vi "pigeon_ver4_1.vi"() -> ()   [LabVIEW 2017]
uses:
  <vilib>/eio/EIONode/EIONode.xnode
  <vilib>/Platform/TimedLoop/XDataNode/XDataNode.xnode
  <vilib>/Platform/TimedLoop/XDataNode/nitl_modes.ctl
  <vilib>/Platform/TimedLoop/XDataNode/XDNodeRunTimeDep.lvlib
  <vilib>/Platform/TimedLoop/XDataNode/wakeup.ctl
  <vilib>/Platform/TimedLoop/XDataNode/timing_clust.ctl
  <vilib>/rvi/DataTransferAndStorage/Container/XNode/niFpgaContainer.xnode
  <vilib>/rvi/eio/common/nirviEmuTemplateMethod_errors.vi
  <vilib>/rvi/Memory/Memory_Emulation/nirvimemoryFastEmulation.vi
  <vilib>/rvi/Memory/Memory_Emulation/nirvimemoryEmulation.vi
  <vilib>/rvi/interface/RandomDataEmulation/nirviRandomDataFpgaReadWriteTemplate.vi
  <vilib>/rvi/Analysis/common/FxpNativeNode/niFpgaFxpNative.xnode
panel:
  out "ramp loop end?":bool=TRUE
  out "ctr":i16
  out "ramp start val":fxp<+,15,15>
  out "Numeric":i16
  in  "analog ramp on":bool
  out "AI2":i16
  in  "Tab Control":enum32{"pigeon"}(tab)
  in  "Emergency Stop":bool
  in  "AO7_pigeon":i16
  in  "AO7":i16
  in  "AO6":i16
  out "trigger AI1":bool
  in  "Tab Control 2":T1(tab)
  in  "square wave  on?":bool
  in  "square wave period":i32
  in  "IGBTswitch":bool caption="IGBT Switch circular"
  in  "Manual Override":bool
  in  "circular coil current":i16(slide) scale=0.0..32768.0
  in  "analog ramp period":i16
  in  "AO4":bool
  in  "analog wave shape":i16(ring) items=["Triangle", "Sawtooth", "Sin", ""]
  in  "analog ramp on  2":bool
  in  "End Current":fxp<+,16,16>
  out "approx rise time [uSec]":u32
  in  "Update Period (uSec)":u32=500
  in  "Points to Add (2^n - 1)":i16=3
  out "FIFO size":i16
  in  "AO0":i16
  in  "AO1":i16
  in  "AO2":i16
  in  "Run program":bool
  in  "halt processor":bool
  out "control flags":i8 format="%b"
  in  "host operation":i16
  in  "address":u16
  in  "data1":u16
  in  "data2":i32
  in  "repeat program":i32
  out "IP address":i16
  out "PMT1":i16=-4740
  out "ReA":i32
  out "RegB":i16
  out "RegC":i16
  out "exttrigger":bool=TRUE
  out "AI1":i16=161
  out "RegD":i16
  in  "AO4":i16
  in  "AO3":i16
  out "Connector0/AI0":i16
  in  "AO5":i16
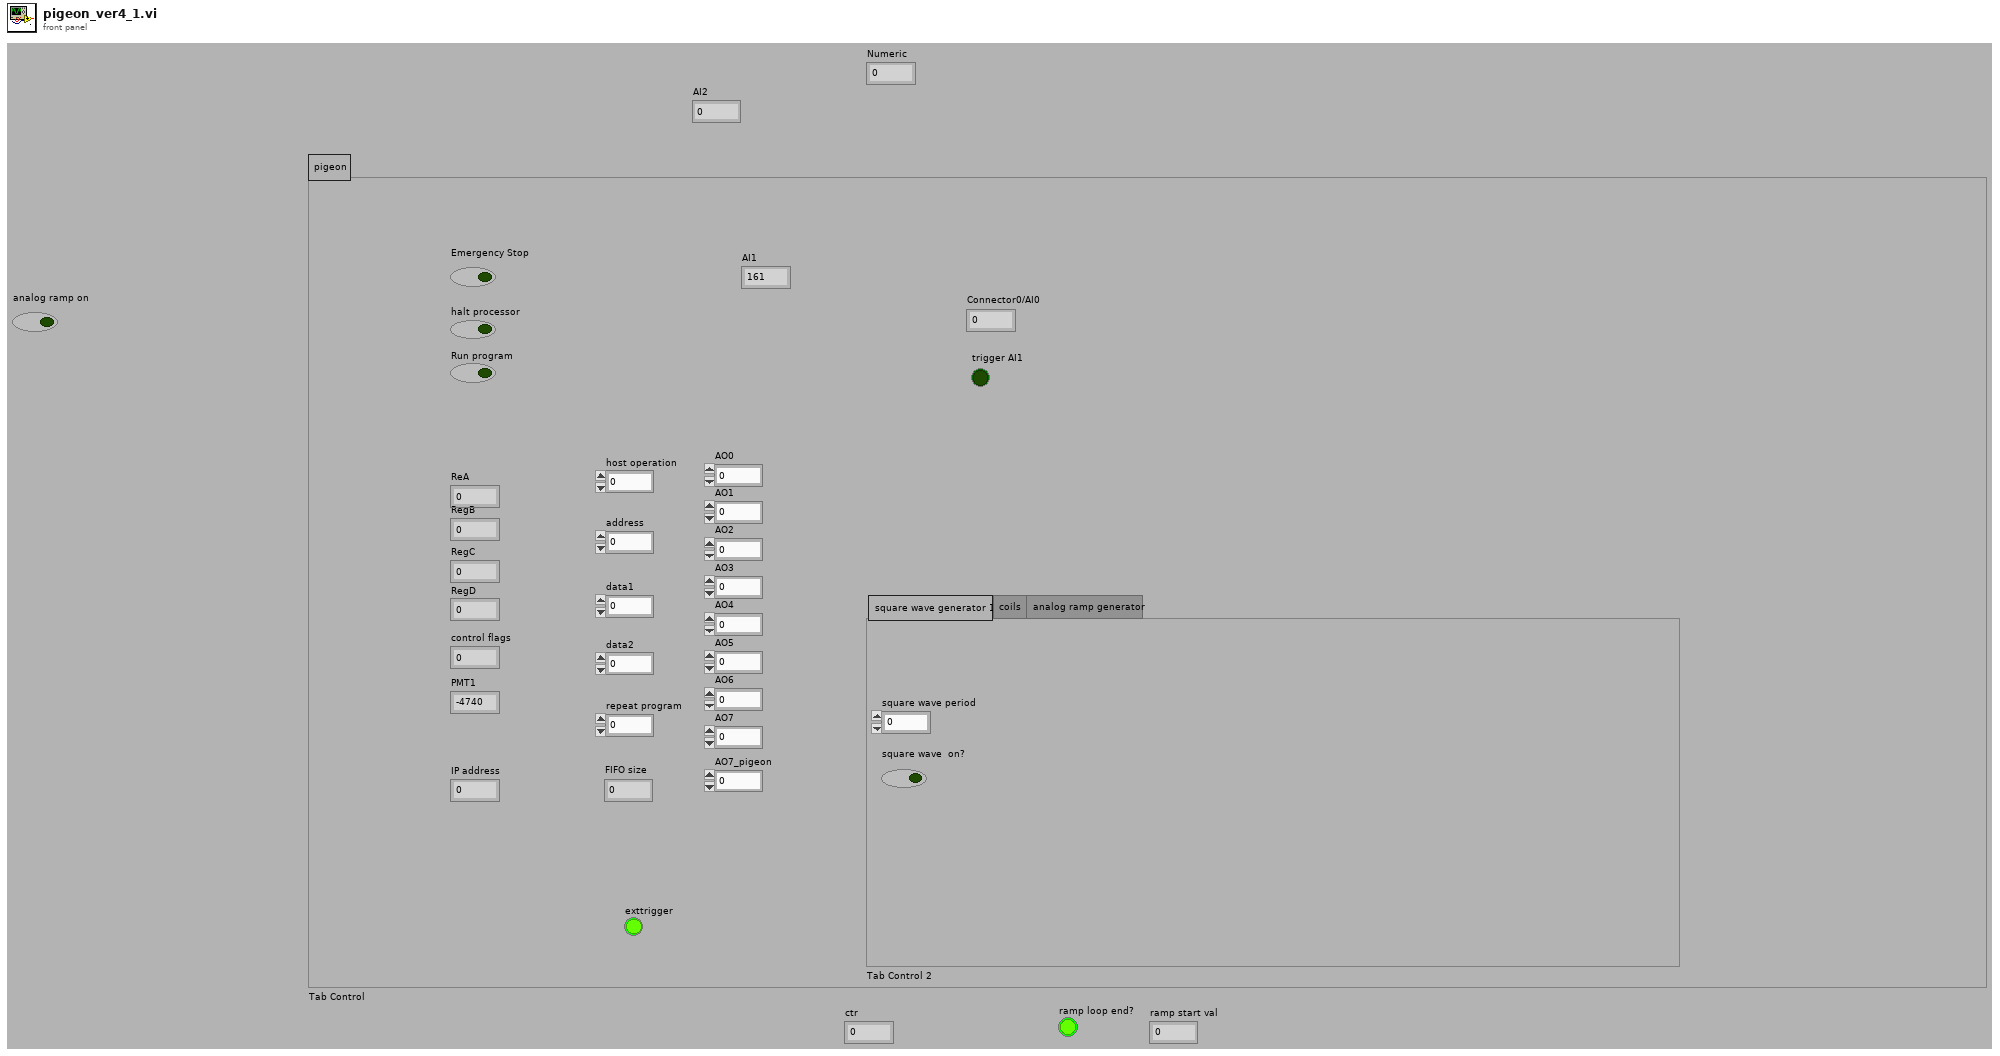
[diagram p1: front panel]
types:
  T1 = enum32{"square wave generator 1", "coils", "analog ramp generator"}
  T2 = typedef "XDNodeRunTimeDep.lvlib/timing_clust.ctl" = cluster{"Expected End [f-1]":u64, "Actual End [f-1]":u64, "Finished Late? [f-1]":bool, "Expected End [i-1]":u64, "Actual End [i-1]":u64, "Finished Late? [i-1]":bool, "Expected Start [i]":u64, "Actual Start [i]":u64, "Expected Start [f]":u64, "Actual Start [f]":u64, "Source Name":string, "Structure Name":string, "Period":i64, "Deadline":i64, "Offset":i64, "Start":i64, "Priority":i32, "Timeout":i32, "Mode":T3, "Wakeup Reason":T4, "Error":errorcluster, "Source Type":string, "Secondary Source Type":string, "Global End Time":u64, "Global Start Time":u64, "Frame Duration":u64, "Iteration Duration":u64, "Assigned CPU":i32, "I/O Scan Engine Mode":u32}
  T3 = typedef "XDNodeRunTimeDep.lvlib/nitl_modes.ctl" = enum32{"No Change", "Process missed periods, maintain original phase", "Discard missed periods, maintain original phase", "Process missed periods, ignore original phase", "Discard missed periods, ignore original phase"}
  T4 = typedef "XDNodeRunTimeDep.lvlib/wakeup.ctl" = enum32{"Normal", "Aborted", "Asynchronous wakeup", "Timing source error", "Timed loop error", "Timeout"}
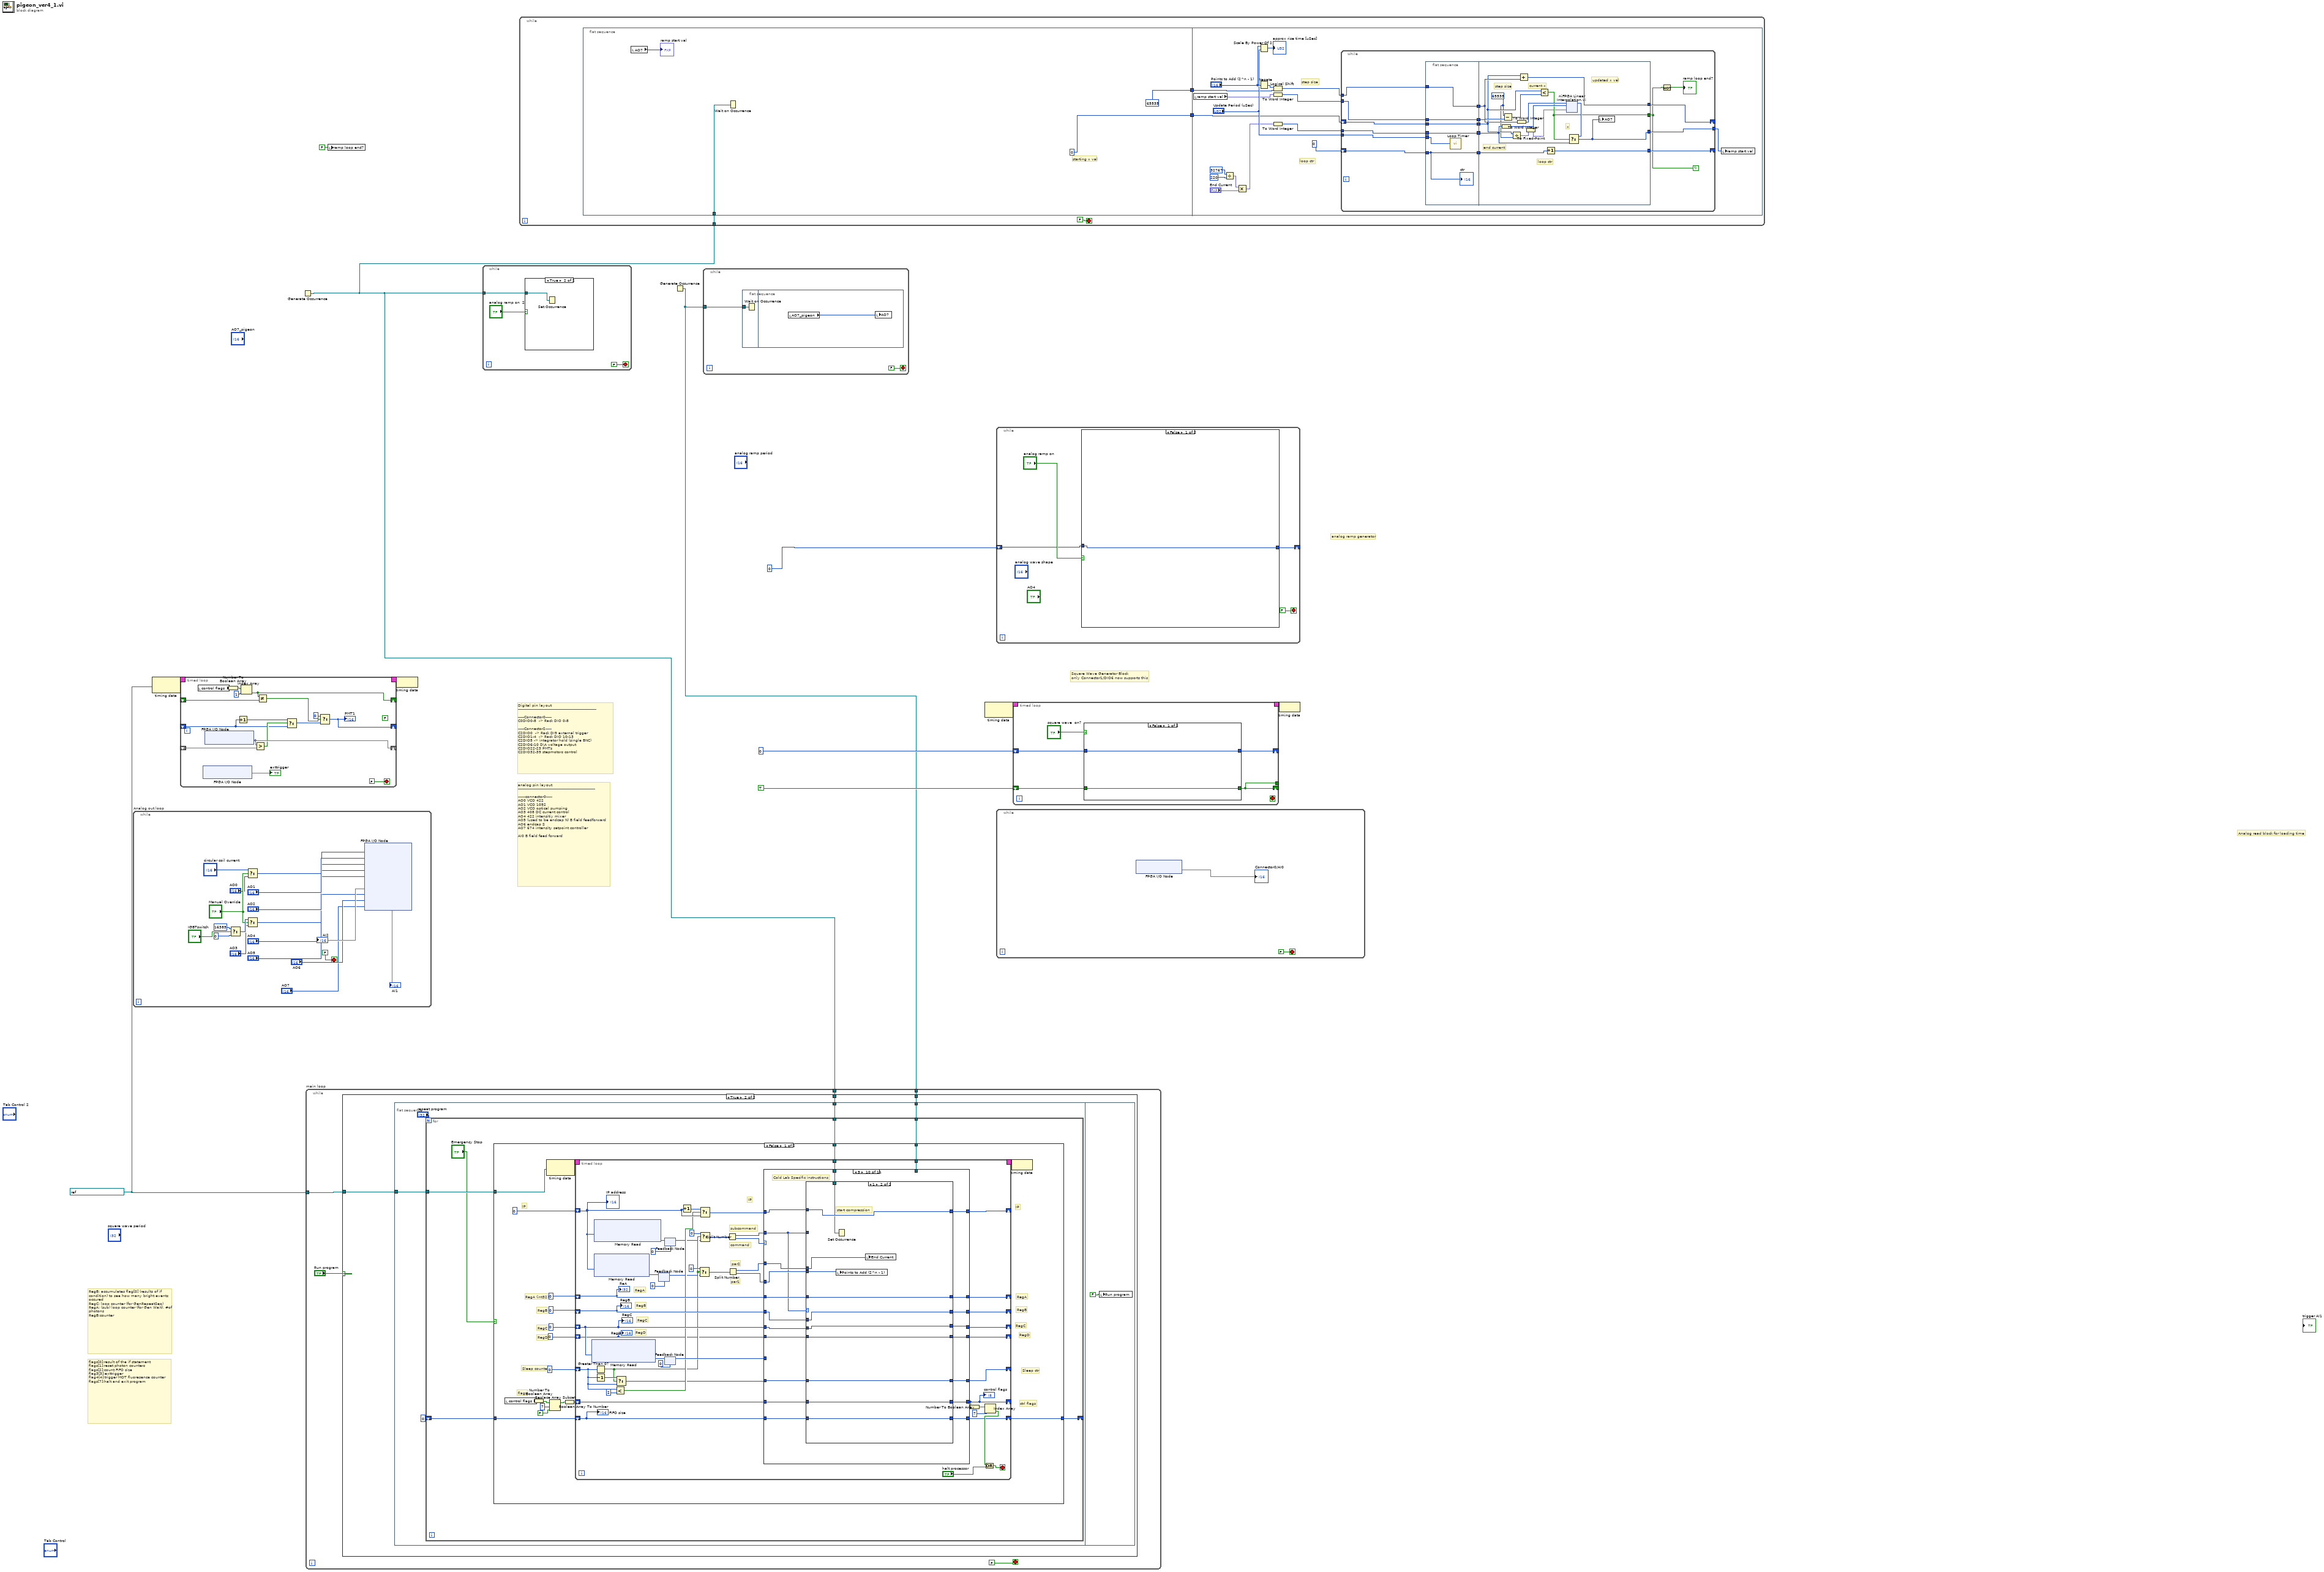
[diagram p0: block diagram]
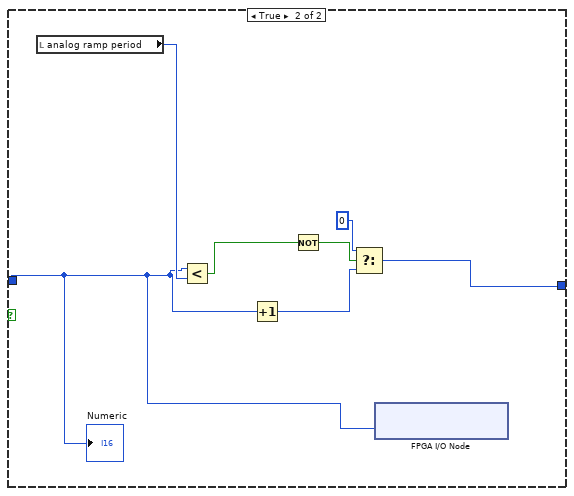
[diagram p3: hidden frame]
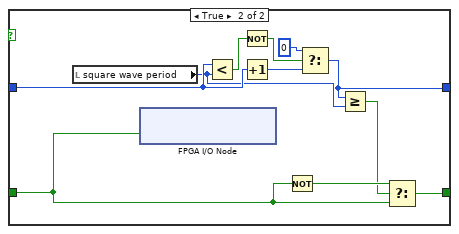
[diagram p4: hidden frame]
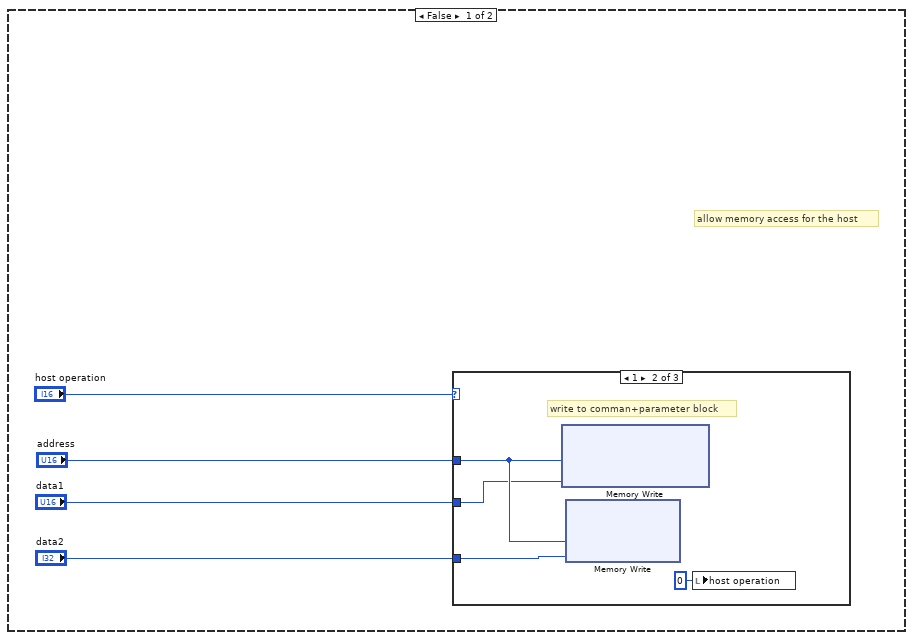
[diagram p5: hidden frame]
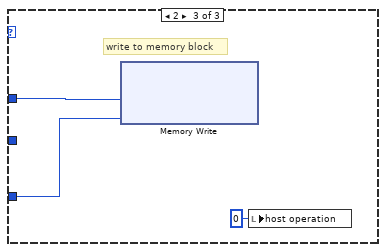
[diagram p7: hidden frame]
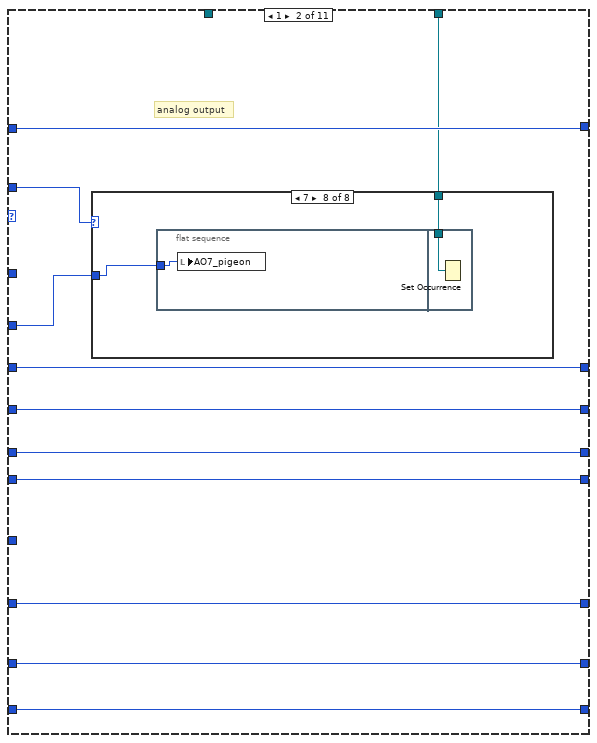
[diagram p9: hidden frame]
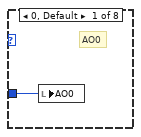
[diagram p10: hidden frame]
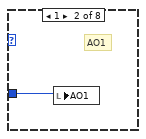
[diagram p11: hidden frame]
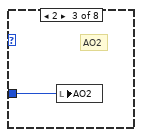
[diagram p12: hidden frame]
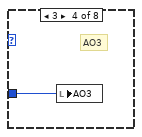
[diagram p13: hidden frame]
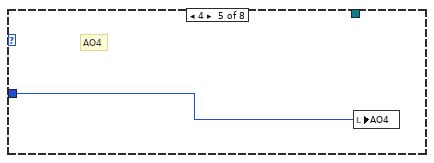
[diagram p14: hidden frame]
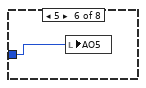
[diagram p15: hidden frame]
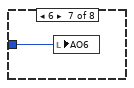
[diagram p16: hidden frame]
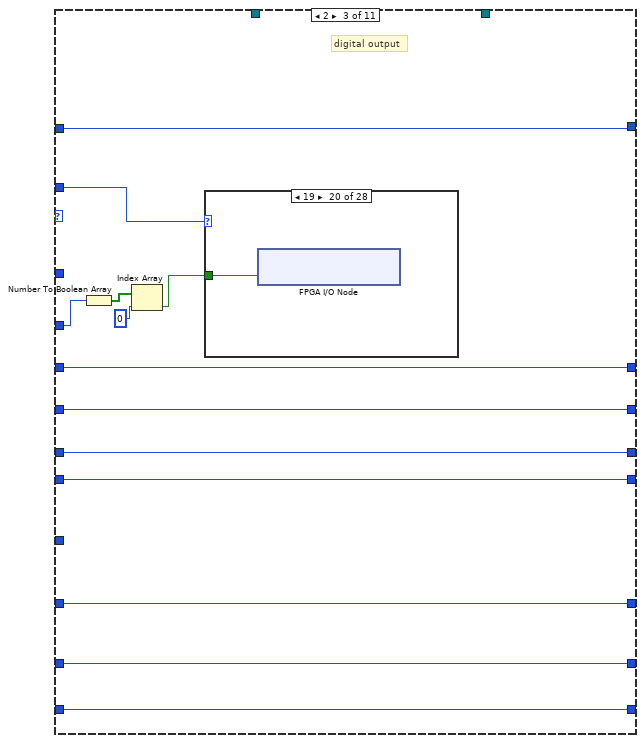
[diagram p17: hidden frame]
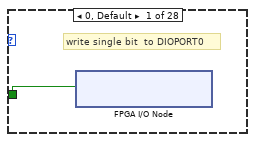
[diagram p18: hidden frame]
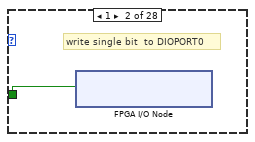
[diagram p19: hidden frame]
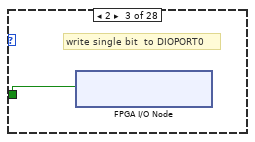
[diagram p20: hidden frame]
diagram:
  w9 = refnum<k21> "40 MHz Onboard Clock" ("FPGA Clock")
  # "analog ramp generator"
  # "Analog read block for loading time"
  # "Square Wave Generator Block\nonly Connector1/DIO6 now supports this"
  # "RegB: accumulates flag[0] (results of if condition) to see how many bright events occured\nRegC: loop counter (for GenRepeatSeq)\nRegA: (sub) loop counter (for Gen Wait), #of     photons \nRegB:counter"
  # "flags[0]:result of the if statement\nflags[1]:reset photon counters\nflags[2]:count FIFO size\nflag3[3]:exttrigger\nflag4[4]:trigger MOT fluoresence counter\nflags[7]:halt and exit program"
  # "Digital pin layout\n----------------------------------------------------------------\n\n-----Connector0-----\nC0DIO0-8  -> Rack DIO 0-8\n\n-----Connector2-----\nC2DIO0  -> Rack DI9 external trigger \nC2DIO1-4  -> Rack DIO 10-13\nC2DIO5 -> integrator hold (single BNC)\nC2DIO6-10 D\\A voltage output\nC2DIO22-23 PMTs\nC2DIO32-39 stepmotors control"
  # "analog pin layout\n---------------------------------------------------------------\n\n------connector0-----\nAO0 VCO 422\nAO1 VCO 1092\nAO2 VCO optical pumping\nAO3 408 DC current control\nAO4 422 intensitiy mixer\nAO5 (used to be endcap N) B field feedforward\nAO6 endcap S\nAO7 674 intensity setpoint controller\n\nAI0 B field feed forward"
  n1 = while "Analog out loop" {
    stop <- FALSE stop-if-true
    n2 = Select(t=i16 16385, s="IGBTswitch", f=i16 0) -> (s? t:f=w20:i16)
    n3 = Select(t="circular coil current", s="Manual Override", f="AO0") -> (s? t:f=w14:i16)
    n4 = Select(t=w20, s="Manual Override", f="AO3") -> (s? t:f=w19:i16)
    n5 = xnode "FPGA I/O Node"("Connector0/AO0"=w14, "Connector0/AO1"="AO1", "Connector0/AO2"="AO2", "Connector0/AO3"=w19, "Connector0/AO4"="AO4", "Connector0/AO5"="AO5", "Connector0/AO6"="AO6", "Connector0/AO7"="AO7") -> ("Connector0/AI1"=→"AI1", "Connector0/AI2"=→"AI2")  [unwired: 10 in, 10 out]
  }
  n6 = node-c288(w9) -> (w11:T2)
  n7 = timed-loop {
    timing: w11 -> [_]
    timing-out: [_] -> w10
    shift-right: [w44] -> _
    shift-left: _ -> [w33]
    shift-right: [w37] -> _
    shift-left: _ -> [w46]
    shift-right: [w39] -> _
    shift-left: _ -> [w40]
    stop <- FALSE stop-if-true
    (unwired) FALSE
    n8 = local read "control flags"() -> (w41:i8)
    n9 = xnode "FPGA I/O Node"() -> ("Connector2/DIO0"=→"exttrigger")  [unwired: 1 in, 1 out]
    n10 = xnode "FPGA I/O Node"() -> ("Connector0/DIO0"=w37)  [unwired: 1 in, 1 out]
    n11 = Number To Boolean Array(number=w41) -> (Boolean array=w42:bool[])
    n12 = Increment(x=w33) -> (x+1=w34:u16)
    n13 = Index Array(array=w42, index=1) -> (element=w39:bool)
    n14 = Greater?(x=w37, y=w46) -> (0:w36:bool)
    n15 = Not Equal?(x=w39, y=w40) -> (x != y?=w31:bool)
    n16 = Select(t=w34, s=w36, f=w33) -> (s? t:f=w45:u16)
    n17 = Select(t=u16 0, s=w31, f=w45) -> (s? t:f=w44:u16)
    "PMT1" <- w44
  }
  n18 = Generate Occurrence() -> (w2:refnum<k4>)
  n19 = local write "ramp loop end?"(FALSE ("ramp loop end?")) -> ()
  n20 = node-c288(w10) -> ()
  n21 = while {
    tunnel: w2 -> [w50]
    stop <- FALSE stop-if-true
    n22 = case shown="True" "analog ramp on  2" {
      tunnel: w50 -> [_ w52]
      frame False {
      }
      frame True {
        n23 = Set Occurrence(w52) -> ()
      }
    }
  }
  n24 = while {
    tunnel: w2 -> [w53]
    stop <- FALSE stop-if-true
    n25 = flat-sequence {
      tunnel: [u16 0] -> w55
      tunnel: [u16 65535 ("x")] -> w54
      tunnel: w53 -> [w57]
      tunnel: w55 -> [w65]
      tunnel: w54 -> [w66]
      frame #0 {
        # "starting x val"
        n26 = local read "AO7"() -> (→"ramp start val":i16)
        n27 = Wait on Occurrence(2:w57) -> ()  [unwired: 2 in, 1 out]
      }
      frame #1 {
        # "loop ctr"
        # "step size"
        n28 = local read "ramp start val"() -> (w62:fxp<+,15,15>)
        n29 = Divide(x=i16 32767, y=i16 220) -> (x/y=w75:fxp<+,16,16>)
        n30 = Multiply(x=w75, y="End Current") -> (x*y=w63:fxp<+,32,32>)
        n31 = Scale By Power Of 2(n="Points to Add (2^n - 1)", x="Update Period (uSec)") -> (x*2^n=→"approx rise time [uSec]":u32)
        n32 = Negate(x="Points to Add (2^n - 1)") -> (-x=w70:i16)
        n33 = Logical Shift(y=w70, x=w66) -> (x << y=w71:u16)
        n34 = To Word Integer(number=w62) -> (16bit integer=w73:i16)
        n35 = To Word Integer(number=w63) -> (16bit integer=w72:i16)
        n36 = while {
          tunnel: w71 -> [w81]
          tunnel: w73 -> [w93]
          tunnel: w72 -> [w92]
          shift-right: [w91] -> _
          shift-left: w65 -> [w80]
          tunnel: "Update Period (uSec)" -> [w90]
          shift-right: [w84] -> _
          shift-left: i16 0 -> [w82]
          tunnel: [w83] -> w64
          stop <- w79 continue-if-true
          n37 = flat-sequence {
            tunnel: w81 -> [w98]
            tunnel: [w98] -> w89
            tunnel: w93 -> [w97]
            tunnel: [w97] -> w88
            tunnel: w92 -> [w96]
            tunnel: [w96] -> w87
            tunnel: w80 -> [w95]
            tunnel: [w95] -> w86
            tunnel: w90 -> [w99]
            tunnel: w82 -> [w94]
            tunnel: [w94] -> w85
            tunnel: w89 -> [w107]
            tunnel: w88 -> [w115]
            tunnel: w87 -> [w105]
            tunnel: w86 -> [w103]
            tunnel: [w108] -> w79
            tunnel: [w109] -> w91
            tunnel: [w111] -> w84
            tunnel: w85 -> [w110]
            tunnel: [w100] -> w83
            frame #0 {
              n38 = call "Loop Timer"("Count(uSec)"=w99) -> ()  [unwired: 1 out]
              "ctr" <- w94
            }
            frame #1 {
              w101 = u16 65535 ("x")
              # "current x"
              # "end current"
              # "x"
              # "loop ctr"
              # "updated x val"
              # "step size"
              n39 = To Word Integer(number=w105) -> (16bit integer=w112:i16)
              n40 = Subtract(x=w101, y=w107) -> (x-y=w106:u16)
              n41 = Divide(x=w103, y=w101) -> (x/y=w102:fxp<+,16,0>)
              n42 = To Word Integer(number=w115) -> (16bit integer=w113:i16)
              n43 = Add(x=w103, y=w107) -> (x+y=w109:u16)
              n44 = To Fixed-Point(number=w102) -> (fixed-point=w104:fxp<+,16,0>)  [unwired: 1 in]
              n45 = Less?(x=w103, y=w106) -> (x < y?=w108:bool)
              n46 = Increment(x=w110) -> (x+1=w111:i16)
              n47 = xnode ("niFPGA Linear Interpolation.vi")("y0"=w113, "y1"=w112, "x"=w104) -> ("y"=w114:i16)
              n48 = Select(t=w114, s=w108, f=w105) -> (s? t:f=w100:i16)
              n49 = local write "AO7"(w100) -> ()
            }
          }
          n50 = Not(x=w79) -> (.not. x?=→"ramp loop end?":bool)
        }
        n51 = local write "ramp start val"(w64) -> ()
      }
    }
  }
  n52 = Generate Occurrence() -> (w1:refnum<k4>)
  n53 = while "main loop" {
    tunnel: w9 -> [w129]
    tunnel: w2 -> [w128]
    tunnel: w1 -> [w127]
    stop <- FALSE ("stop") stop-if-true
    n54 = case shown="True" "Run program" {
      tunnel: w129 -> [_ w145]
      tunnel: w128 -> [_ w144]
      tunnel: w127 -> [_ w143]
      frame False {
        # "allow memory access for the host"
        n55 = case shown="1" "host operation" {
          tunnel: "address" -> [_ w137 w142]
          tunnel: "data1" -> [_ w136 _]
          tunnel: "data2" -> [_ w139 w140]
          frame 0, Default {
          }
          frame 1 {
            # "write to comman+parameter block"
            n56 = xnode ("Memory Write")("Address"=w137, "Data"=w136) -> ()  [unwired: 1 in, 1 out]
            n57 = xnode ("Memory Write")("Address"=w137, "Data"=w139) -> ()  [unwired: 1 in, 1 out]
            n58 = local write "host operation"(i16 0 ("host operation")) -> ()
          }
          frame 2 {
            # "write to memory block"
            n59 = xnode ("Memory Write")("Address"=w142, "Data"=w140) -> ()  [unwired: 1 in, 1 out]
            n60 = local write "host operation"(i16 0 ("host operation")) -> ()
          }
        }
      }
      frame True {
        n61 = flat-sequence {
          tunnel: w145 -> [w149]
          tunnel: w144 -> [w147]
          tunnel: w143 -> [w146]
          frame #0 {
            n62 = for {
              N: "repeat program" -> [_]
              tunnel: w149 -> [w156]
              shift-right: [w154] -> _
              shift-left: i16 0 -> [w155]
              tunnel: w147 -> [w153]
              tunnel: w146 -> [w152]
              n63 = case shown="False" "Emergency Stop" {
                tunnel: w156 -> [w169 _]
                tunnel: w155 -> [w161 w633]
                tunnel: [w160 w633] -> w154
                tunnel: w153 -> [w158 _]
                tunnel: w152 -> [w157 _]
                frame False {
                  # "ctrl flags"
                  # "Sleep ctr"
                  # "RegD"
                  # "RegD"
                  # "Sleep counter"
                  # "flags"
                  # "RegC"
                  # "RegB"
                  # "RegA"
                  # "RegC"
                  # "RegB"
                  # "RegA (int32)"
                  # "IP"
                  # "IP"
                  n64 = local read "control flags"() -> (w164:i8)
                  n65 = Number To Boolean Array(number=w164) -> (Boolean array=w168:bool[])
                  n66 = node-c288(w169) -> (w175:T2)
                  n67 = Replace Array Subset(array=w168, new element=FALSE ("new element/subarray"), index=7) -> (w166:bool[])
                  n68 = Boolean Array To Number(Boolean array=w166) -> (number=w167:u8)
                  n69 = timed-loop {
                    timing: w175 -> [_]
                    timing-out: [_] -> w174
                    shift-right: [w212] -> _
                    shift-left: i16 0 -> [w195]
                    shift-right: [w208] -> _
                    shift-left: 0 -> [w204]
                    shift-right: [w220] -> _
                    shift-left: i16 0 -> [w211]
                    shift-right: [w219] -> _
                    shift-left: i16 0 -> [w203]
                    shift-right: [w209] -> _
                    shift-left: w167 -> [w210]
                    shift-right: [w202] -> _
                    shift-left: i16 0 -> [w193]
                    shift-right: [w184] -> w160
                    shift-left: w161 -> [w183]
                    shift-right: [w181] -> _
                    shift-left: i16 0 -> [w182]
                    tunnel: w158 -> [w177]
                    tunnel: w157 -> [w176]
                    stop <- w215 stop-if-true
                    # "RegD"
                    # "IP"
                    # "RegC"
                    # "RegB"
                    # "RegA"
                    # "par1"
                    # "par2"
                    # "subcommand"
                    # "command"
                    n70 = xnode ("Memory Read")("Address"=w203) -> ("Data"=w207:i16)  [unwired: 2 in, 2 out]
                    n71 = xnode ("Memory Read")("Address"=w195) -> ("Data"=w190:u16)  [unwired: 1 in, 1 out]
                    n72 = xnode ("Memory Read")("Address"=w195) -> ("Data"=w186:i32)  [unwired: 1 in, 1 out]
                    n73 = Greater Than 0?(x=w193) -> (x > 0?=w188:bool)
                    n74 = Decrement(x=w193) -> (x-1=w194:u32)
                    n75 = Less?(x=w193, y=u32 2) -> (x < y?=w192:bool)
                    n76 = Select(t=w194, s=w188, f=w193) -> (s? t:f=w191:u32)
                    n77 = feedback-in #1(w186) -> ()
                    n78 = feedback #1(u32 0 ("Data")) -> (w185:u32)
                    n79 = feedback-in #2(w207) -> ()
                    n80 = feedback #2(0) -> (w206:i32)
                    n81 = feedback-in #3(w190) -> ()
                    n82 = feedback #3(u16 0 ("Data")) -> (w187:u16)
                    n83 = Increment(x=w195) -> (x+1=w196:u16)
                    n84 = Select(t=0, s=w188, f=w185) -> (s? t:f=w199:u32)
                    n85 = Select(t=w196, s=w192, f=w195) -> (s? t:f=w201:u16)
                    n86 = Select(t=u16 0, s=w188, f=w187) -> (s? t:f=w200:u16)
                    n87 = Split Number(x=w200) -> (hi(x)=w221:u8, lo(x)=w222:u8)
                    n88 = Split Number(x=w199) -> (hi(x)=w213:u16, lo(x)=w214:u16)
                    n89 = case shown="9" w222 {
                      tunnel: w214 -> [_ w240 w257 _ w337 w457 w531 _ _ w591 _]
                      tunnel: w213 -> [_ _ _ _ w330 w456 w530 _ _ w592 _]
                      tunnel: w221 -> [_ w241 w265 w304 w338 w461 _ w549 _ w573 _]
                      tunnel: w204 -> [w230 w239 w264 w296 w336 w458 w535 w553 w569 w590 w620]
                      tunnel: [w230 w239 w264 w296 w333 w458 w535 w553 w569 w589 w620] -> w208
                      tunnel: w211 -> [w229 w238 w263 w295 w335 w459 w536 w552 w572 w588 w621]
                      tunnel: w203 -> [w228 w237 w262 w302 w334 w460 w537 w551 w571 w586 w622]
                      tunnel: [w229 w238 w263 w294 w332 w459 w536 w552 w572 w587 w621] -> w220
                      tunnel: [w228 w237 w262 w302 w331 w460 w537 w551 w571 w585 w622] -> w219
                      tunnel: [w226 w236 w261 w303 w326 w464 w529 w555 w570 w575 w619] -> w212
                      tunnel: w201 -> [w226 w236 w261 w303 w327 w464 _ w555 w570 w576 w619]
                      tunnel: [w227 w235 w260 w300 w328 w463 w528 w544 w566 w579 w625] -> w209
                      tunnel: w210 -> [w227 w235 w260 w301 w329 w462 w528 w543 w565 w580 w625]
                      tunnel: w206 -> [_ _ _ _ w320 w455 _ _ _ _ _]
                      tunnel: w191 -> [w225 w234 w255 w299 w325 w454 w527 w541 w562 w582 w626]
                      tunnel: [w225 w234 w255 w299 w324 w454 w527 w541 w562 w581 w626] -> w202
                      tunnel: w183 -> [w224 w233 w254 w298 w323 w453 w526 w540 w561 w577 w624]
                      tunnel: [w224 w233 w254 w298 w323 w453 w526 w539 w561 w578 w624] -> w184
                      tunnel: w182 -> [w223 w232 w253 w297 w322 w452 w525 w538 w560 w584 w623]
                      tunnel: [w223 w232 w253 w297 w321 w452 w525 w538 w560 w583 w623] -> w181
                      tunnel: w177 -> [_ _ _ _ _ _ _ _ _ w574 _]
                      tunnel: w176 -> [_ w231 _ _ _ _ _ _ _ _ _]
                      frame 0, Default {
                      }
                      frame 1 {
                        # "analog output"
                        n90 = case shown="7" w241 {
                          tunnel: w240 -> [w242 w243 w244 w245 w246 w247 w248 w250]
                          tunnel: w231 -> [_ _ _ _ _ _ _ w249]
                          frame 0, Default {
                            # "AO0"
                            n91 = local write "AO0"(w242) -> ()
                          }
                          frame 1 {
                            # "AO1"
                            n92 = local write "AO1"(w243) -> ()
                          }
                          frame 2 {
                            # "AO2"
                            n93 = local write "AO2"(w244) -> ()
                          }
                          frame 3 {
                            # "AO3"
                            n94 = local write "AO3"(w245) -> ()
                          }
                          frame 4 {
                            # "AO4"
                            n95 = local write "AO4"(w246) -> ()
                          }
                          frame 5 {
                            n96 = local write "AO5"(w247) -> ()
                          }
                          frame 6 {
                            n97 = local write "AO6"(w248) -> ()
                          }
                          frame 7 {
                            n98 = flat-sequence {
                              tunnel: w250 -> [w251]
                              tunnel: w249 -> [w252]
                              frame #0 {
                                n99 = local write "AO7_pigeon"(w251) -> ()
                              }
                              frame #1 {
                                n100 = Set Occurrence(w252) -> ()
                              }
                            }
                          }
                        }
                      }
                      frame 2 {
                        # "digital output"
                        n101 = Number To Boolean Array(number=w257) -> (Boolean array=w258:bool[])
                        n102 = Index Array(array=w258, index=0) -> (element=w256:bool)
                        n103 = case shown="19" w265 {
                          tunnel: w256 -> [w266 w267 w268 w269 w270 w271 w272 w273 w274 w275 w276 w277 w278 w279 w280 w281 w282 w283 w284 w285 w286 w287 w288 w289 w290 w291 w292 w293]
                          frame 0, Default {
                            # "write single bit  to DIOPORT0"
                            n104 = xnode "FPGA I/O Node"("Connector1/DIO0"=w266) -> ()  [unwired: 1 in, 1 out]
                          }
                          frame 1 {
                            # "write single bit  to DIOPORT0"
                            n105 = xnode "FPGA I/O Node"("Connector1/DIO1"=w267) -> ()  [unwired: 1 in, 1 out]
                          }
                          frame 2 {
                            # "write single bit  to DIOPORT0"
                            n106 = xnode "FPGA I/O Node"("Connector1/DIO2"=w268) -> ()  [unwired: 1 in, 1 out]
                          }
                          frame 3 {
                            # "write single bit  to DIOPORT0"
                            n107 = xnode "FPGA I/O Node"("Connector1/DIO3"=w269) -> ()  [unwired: 1 in, 1 out]
                          }
                          frame 4 {
                            # "write single bit  to DIOPORT0"
                            n108 = xnode "FPGA I/O Node"("Connector1/DIO4"=w270) -> ()  [unwired: 1 in, 1 out]
                          }
                          frame 5 {
                            # "write single bit  to DIOPORT0"
                            n109 = xnode "FPGA I/O Node"("Connector1/DIO5"=w271) -> ()  [unwired: 1 in, 1 out]
                          }
                          frame 6 {
                            # "write single bit  to DIOPORT0"
                            n110 = xnode "FPGA I/O Node"("Connector1/DIO6"=w272) -> ()  [unwired: 1 in, 1 out]
                          }
                          frame 7 {
                            # "write single bit  to DIOPORT0"
                            n111 = xnode "FPGA I/O Node"("Connector1/DIO7"=w273) -> ()  [unwired: 1 in, 1 out]
                          }
                          frame 8 {
                            # "write single bit  to DIOPORT0"
                            n112 = xnode "FPGA I/O Node"("Connector1/DIO8"=w274) -> ()  [unwired: 1 in, 1 out]
                          }
                          frame 9 {
                            n113 = xnode "FPGA I/O Node"("Connector1/DIO9"=w275) -> ()  [unwired: 1 in, 1 out]
                          }
                          frame 10 {
                            n114 = xnode "FPGA I/O Node"("Connector1/DIO10"=w276) -> ()  [unwired: 1 in, 1 out]
                          }
                          frame 11 {
                            n115 = xnode "FPGA I/O Node"("Connector1/DIO11"=w277) -> ()  [unwired: 1 in, 1 out]
                          }
                          frame 12 {
                            n116 = xnode "FPGA I/O Node"("Connector1/DIO12"=w278) -> ()  [unwired: 1 in, 1 out]
                          }
                          frame 13 {
                            n117 = xnode "FPGA I/O Node"("Connector1/DIO13"=w279) -> ()  [unwired: 1 in, 1 out]
                          }
                          frame 14 {
                            n118 = xnode "FPGA I/O Node"("Connector1/DIO14"=w280) -> ()  [unwired: 1 in, 1 out]
                          }
                          frame 15 {
                            n119 = xnode "FPGA I/O Node"("Connector1/DIO15"=w281) -> ()  [unwired: 1 in, 1 out]
                          }
                          frame 16 {
                            n120 = xnode "FPGA I/O Node"("Connector1/DIO16"=w282) -> ()  [unwired: 1 in, 1 out]
                          }
                          frame 17 {
                            n121 = xnode "FPGA I/O Node"("Connector1/DIO17"=w283) -> ()  [unwired: 1 in, 1 out]
                          }
                          frame 18 {
                            n122 = xnode "FPGA I/O Node"("Connector1/DIO18"=w284) -> ()  [unwired: 1 in, 1 out]
                          }
                          frame 19 {
                            n123 = xnode "FPGA I/O Node"("Connector1/DIO19"=w285) -> ()  [unwired: 1 in, 1 out]
                          }
                          frame 20 {
                            n124 = xnode "FPGA I/O Node"("Connector2/DIO12"=w286) -> ()  [unwired: 1 in, 1 out]
                          }
                          frame 21 {
                            n125 = xnode "FPGA I/O Node"("Connector2/DIO17"=w287) -> ()  [unwired: 1 in, 1 out]
                          }
                          frame 22 {
                            n126 = xnode "FPGA I/O Node"("Connector2/DIO19"=w288) -> ()  [unwired: 1 in, 1 out]
                          }
                          frame 23 {
                            n127 = xnode "FPGA I/O Node"("Connector2/DIO18"=w289) -> ()  [unwired: 1 in, 1 out]
                          }
                          frame 24 {
                            n128 = xnode "FPGA I/O Node"("Connector2/DIO21"=w290) -> ()  [unwired: 1 in, 1 out]
                          }
                          frame 25 {
                            n129 = xnode "FPGA I/O Node"("Connector2/DIO24"=w291) -> ()  [unwired: 1 in, 1 out]
                          }
                          frame 26 {
                            n130 = xnode "FPGA I/O Node"("Connector2/DIO25"=w292) -> ()  [unwired: 1 in, 1 out]
                          }
                          frame 27 {
                            n131 = xnode "FPGA I/O Node"("Connector2/DIO20"=w293) -> ()  [unwired: 1 in, 1 out]
                          }
                        }
                      }
                      frame 3 {
                        # "photon counting"
                        n132 = case shown="3" w304 {
                          tunnel: [w305 w307 w319] -> w294
                          tunnel: w295 -> [w305 w308 w319]
                          tunnel: w301 -> [w306 w310 w317]
                          tunnel: [w306 w310 w316] -> w300
                          frame 2, Default {
                          }
                          frame 1 {
                            # "PMT1"
                            n133 = local read "PMT1"() -> (w309:i16)
                            n134 = Add(x=w309, y=w308) -> (x+y=w307:u16)
                          }
                          frame 3 {
                            # "Reset  photon counter"
                            # "make a Not gate of flag(1)"
                            n135 = Number To Boolean Array(number=w317) -> (Boolean array=w314:bool[])
                            n136 = Index Array(array=w314, index=1) -> (element=w312:bool)
                            n137 = Not(x=w312) -> (.not. x?=w311:bool)
                            n138 = Replace Array Subset(array=w314, new element=w311, index=1) -> (w315:bool[])
                            n139 = Boolean Array To Number(Boolean array=w315) -> (number=w316:u8)
                          }
                        }
                      }
                      frame 4 {
                        # "registers operation"
                        n140 = case shown="7" w338 {
                          tunnel: w337 -> [w344 w354 w361 _ _ _ _ w403 _ _ w430 w443]
                          tunnel: w336 -> [_ w353 w360 w367 w375 w383 w387 w408 w419 w425 w435 w448]
                          tunnel: w335 -> [w347 _ w359 w366 w377 w382 w395 w407 w418 w421 w433 w446]
                          tunnel: w334 -> [w346 w352 _ w369 w376 _ w388 w406 w417 w424 w434 w447]
                          tunnel: [w343 w353 w360 w367 w374 w383 w387 w408 w419 w425 w435 w448] -> w333
                          tunnel: [w347 w354 w359 w366 w377 w382 w394 w407 w418 w423 w433 w446] -> w332
                          tunnel: [w346 w352 w361 w368 w376 w382 w388 w406 w417 w424 w434 w447] -> w331
                          tunnel: w330 -> [w345 _ _ _ _ _ _ w404 _ _ _ w442]
                          tunnel: w329 -> [w342 w351 w358 w365 w373 w381 w389 w405 w416 w428 w438 w451]
                          tunnel: [w342 w351 w358 w365 w373 w381 w389 w405 w416 w428 w438 w451] -> w328
                          tunnel: w327 -> [w341 w350 w357 w364 w372 w380 w386 w397 w411 w427 w437 w450]
                          tunnel: [w341 w350 w357 w364 w372 w380 w386 w400 w414 w427 w437 w450] -> w326
                          tunnel: w325 -> [w340 w349 w356 w363 w371 w379 w385 _ _ w426 w436 w449]
                          tunnel: [w340 w349 w356 w363 w371 w379 w385 w401 w409 w426 w436 w449] -> w324
                          tunnel: w322 -> [w339 w348 w355 w362 w370 w378 w384 w396 w410 w420 _ w441]
                          tunnel: [w339 w348 w355 w362 w370 w378 w384 w396 w410 w420 w431 w440] -> w321
                          tunnel: w320 -> [_ _ _ _ _ _ _ _ w409 _ _ _]
                          frame 0, Default {
                            # "Set par1,2 to RegA"
                            n141 = Join Numbers(hi=w345, lo=w344) -> ((hi.lo)=w343:u32)
                          }
                          frame 1 {
                            # "Set par1 to RegB"
                          }
                          frame 2 {
                            # "Set par1 to RegC"
                          }
                          frame 3 {
                            # "increase RegC by 1"
                            n142 = Increment(x=w369) -> (x+1=w368:u16)
                          }
                          frame 4 {
                            # "increase RegA by 1"
                            n143 = Increment(x=w375) -> (x+1=w374:u32)
                          }
                          frame 5 {
                            # "Set regC to regB"
                          }
                          frame 6 {
                            # "regB<-regB+flags[0]"
                            n144 = Number To Boolean Array(number=w389) -> (Boolean array=w393:bool[])
                            n145 = Index Array(array=w393, index=0) -> (element=w391:bool)
                            n146 = Boolean To (0,1)(Boolean=w391) -> (0, 1=w390:i16)
                            n147 = Add(x=w390, y=w395) -> (x+y=w394:u16)
                          }
                          frame 7 {
                            # "Sleep counter = [par1 par2]"
                            n148 = Join Numbers(hi=w404, lo=w403) -> ((hi.lo)=w401:u32)
                            n149 = Greater?(x=w401, y=u32 0) -> (0:w399:bool)
                            n150 = Decrement(x=w397) -> (x-1=w398:u16)
                            n151 = Select(t=w398, s=w399, f=w397) -> (s? t:f=w400:u16)
                          }
                          frame 11 {
                            # "Sleep counter =par1* memory Block[RegC]"
                            n152 = Greater?(x=w409, y=u32 0) -> (0:w413:bool)
                            n153 = Decrement(x=w411) -> (x-1=w412:u16)
                            n154 = Select(t=w412, s=w413, f=w411) -> (s? t:f=w414:u16)
                          }
                          frame 8 {
                            # "RegB=RegB+ RegA(lo)"
                            n155 = Split Number(x=w425) -> (lo(x)=w422:u16)  [unwired: 1 out]
                            n156 = Add(x=w422, y=w421) -> (x+y=w423:u16)
                          }
                          frame 9 {
                            # "RegD<-AI1+par1"
                            n157 = To Word Integer(number=w430) -> (16bit integer=w429:i16)
                            n158 = local read "AI1"() -> (w432:i16)
                            n159 = Add(x=w429, y=w432) -> (x+y=w431:i16)
                          }
                          frame 10 {
                            # "RegD<-RegD*2^par1*par2"
                            n160 = To Word Integer(number=w442) -> (16bit integer=w444:i16)
                            n161 = To Word Integer(number=w443) -> (16bit integer=w445:i16)
                            n162 = Multiply(x=w444, y=w441) -> (x*y=w439:i16)
                            n163 = Scale By Power Of 2(n=w445, x=w439) -> (x*2^n=w440:i16)
                          }
                        }
                      }
                      frame 5 {
                        # "If statement"
                        n164 = case shown="4" w461 {
                          tunnel: [w474 w482 w490 w498 w508 w511 w519] -> w463
                          tunnel: w462 -> [w473 w481 w489 w497 w507 w512 w520]
                          tunnel: w456 -> [w467 _ _ _ _ _ _]
                          tunnel: w460 -> [_ _ w485 w492 _ _ _]
                          tunnel: w459 -> [_ w476 _ w491 _ _ _]
                          tunnel: w458 -> [w468 _ _ _ _ w509 w517]
                          tunnel: w457 -> [w466 w475 w484 _ _ w510 _]
                          tunnel: w455 -> [_ _ _ _ _ _ w524]
                          frame 0, Default {
                            # "The if regA =  [par1,par2]"
                            n165 = Number To Boolean Array(number=w473) -> (Boolean array=w471:bool[])
                            n166 = Join Numbers(hi=w467, lo=w466) -> ((hi.lo)=w465:u32)
                            n167 = Equal?(x=w465, y=w468) -> (x = y?=w469:bool)
                            n168 = Replace Array Subset(array=w471, new element=w469, index=0) -> (w470:bool[])
                            n169 = Boolean Array To Number(Boolean array=w470) -> (number=w474:u8)
                          }
                          frame 1 {
                            # "The if  regB >  par1"
                            n170 = Number To Boolean Array(number=w481) -> (Boolean array=w479:bool[])
                            n171 = Greater?(x=w476, y=w475) -> (0:w477:bool)
                            n172 = Replace Array Subset(array=w479, new element=w477, index=0) -> (w478:bool[])
                            n173 = Boolean Array To Number(Boolean array=w478) -> (number=w482:u8)
                          }
                          frame 2 {
                            # "The if  regC=  par1"
                            n174 = Number To Boolean Array(number=w489) -> (Boolean array=w487:bool[])
                            n175 = Equal?(x=w484, y=w485) -> (x = y?=w483:bool)
                            n176 = Replace Array Subset(array=w487, new element=w483, index=0) -> (w486:bool[])
                            n177 = Boolean Array To Number(Boolean array=w486) -> (number=w490:u8)
                          }
                          frame 3 {
                            # "The if  regB> regC"
                            n178 = Number To Boolean Array(number=w497) -> (Boolean array=w495:bool[])
                            n179 = Greater?(x=w491, y=w492) -> (0:w493:bool)
                            n180 = Replace Array Subset(array=w495, new element=w493, index=0) -> (w494:bool[])
                            n181 = Boolean Array To Number(Boolean array=w494) -> (number=w498:u8)
                          }
                          frame 4 {
                            w503 = 3 ("index")
                            # "external trigger rising edge"
                            n182 = Number To Boolean Array(number=w507) -> (Boolean array=w504:bool[])
                            n183 = local read "exttrigger"() -> (w500:bool)
                            n184 = Index Array(array=w504, index=w503) -> (element=w502:bool)
                            n185 = Not(x=w502) -> (.not. x?=w501:bool)
                            n186 = And(x=w500, y=w501) -> (x .and. y?=w499:bool)
                            n187 = Replace Array Subset(array=w504, new element #1=w499, index #1=0 ("index"), new element #2=w500, index #2=w503) -> (w505:bool[])
                            n188 = Boolean Array To Number(Boolean array=w505) -> (number=w508:u8)
                          }
                          frame 5 {
                            # "The if  regA >  par1"
                            n189 = Number To Boolean Array(number=w512) -> (Boolean array=w515:bool[])
                            n190 = Greater?(x=w509, y=w510) -> (0:w513:bool)
                            n191 = Replace Array Subset(array=w515, new element=w513, index=0) -> (w514:bool[])
                            n192 = Boolean Array To Number(Boolean array=w514) -> (number=w511:u8)
                          }
                          frame 6 {
                            # "The if  regA == memoryBlock(regC)"
                            n193 = Number To Boolean Array(number=w520) -> (Boolean array=w522:bool[])
                            n194 = Equal?(x=w517, y=w524) -> (x = y?=w518:bool)
                            n195 = Replace Array Subset(array=w522, new element=w518, index=0) -> (w521:bool[])
                            n196 = Boolean Array To Number(Boolean array=w521) -> (number=w519:u8)
                          }
                        }
                      }
                      frame 6 {
                        # "condition (flags[0]) goto\nuse par1=par2 for normal goto"
                        n197 = Number To Boolean Array(number=w528) -> (Boolean array=w534:bool[])
                        n198 = Index Array(array=w534, index=0) -> (element=w532:bool)
                        n199 = Select(t=w531, s=w532, f=w530) -> (s? t:f=w529:u16)
                      }
                      frame 7 {
                        w542 = 2 ("index")
                        # "make a Not gate of flag(2)"
                        # "push  to FIFO"
                        n200 = case shown="4" w549 {
                          tunnel: w553 -> [w556 _ _ _]
                          tunnel: w552 -> [_ w557 _ _]
                          tunnel: w551 -> [_ _ w558 _]
                          tunnel: [w556 w557 w558 w559] -> w550
                          frame 0, Default {
                            # "push RegA"
                          }
                          frame 1 {
                            # "push RegB"
                          }
                          frame 2 {
                            # "push RegC"
                          }
                          frame 4 {
                            n201 = local read "AI1"() -> (w559:i16)
                          }
                        }
                        n202 = Number To Boolean Array(number=w543) -> (Boolean array=w547:bool[])
                        n203 = Index Array(array=w547, index=w542) -> (element=w546:bool)
                        n204 = Not(x=w546) -> (.not. x?=w545:bool)
                        n205 = Replace Array Subset(array=w547, new element=w545, index=w542) -> (w548:bool[])
                        n206 = Increment(x=w540) -> (x+1=w539:i16)
                        n207 = Boolean Array To Number(Boolean array=w548) -> (number=w544:u8)
                        n208 = xnode ("FIFO Write")("Element"=w550, "Timeout"=0) -> ()  [unwired: 1 in, 2 out]
                      }
                      frame 8 {
                        # "Stop and reset program"
                        n209 = Number To Boolean Array(number=w565) -> (Boolean array=w568:bool[])
                        n210 = Replace Array Subset(array=w568, new element=TRUE ("new element/subarray"), index=7) -> (w567:bool[])
                        n211 = Boolean Array To Number(Boolean array=w567) -> (number=w566:u8)
                      }
                      frame 9 {
                        # "Cold Lab Specific instructions"
                        n212 = case shown="1" w573 {
                          tunnel: w592 -> [w605 w610]
                          tunnel: w591 -> [w604 w609]
                          tunnel: w590 -> [w601 w611]
                          tunnel: [w601 w611] -> w589
                          tunnel: w588 -> [w600 w612]
                          tunnel: [w600 w612] -> w587
                          tunnel: w586 -> [w599 w613]
                          tunnel: [w599 w613] -> w585
                          tunnel: w584 -> [w598 w614]
                          tunnel: [w598 w614] -> w583
                          tunnel: w582 -> [w597 w615]
                          tunnel: [w597 w615] -> w581
                          tunnel: w580 -> [w596 w616]
                          tunnel: [w596 w616] -> w579
                          tunnel: [w595 w617] -> w578
                          tunnel: w577 -> [w595 w617]
                          tunnel: w576 -> [w594 w608]
                          tunnel: [w594 w608] -> w575
                          tunnel: w574 -> [_ w607]
                          tunnel: w573 -> [w593 _]
                          frame 0, Default {
                            # "Run Square wave generator"
                            n213 = Greater?(x=w593, y=u8 0) -> (0:w602:bool)
                            n214 = Join Numbers(hi=w605, lo=w604) -> ((hi.lo)=w606:u32)
                            n215 = local write "square wave  on?"(w602) -> ()
                            n216 = local write "square wave period"(w606) -> ()
                          }
                          frame 1 {
                            # "start compression"
                            n217 = Set Occurrence(w607) -> ()
                            n218 = local write "Points to Add (2^n - 1)"(w609) -> ()
                            n219 = local write "End Current"(w610) -> ()
                          }
                        }
                      }
                      frame 10 {
                        n220 = local write "trigger AI1"(TRUE) -> ()
                      }
                    }
                    "control flags" <- w209
                    n221 = Number To Boolean Array(number=w209) -> (Boolean array=w218:bool[])
                    n222 = Index Array(array=w218, index=7) -> (element=w216:bool)
                    n223 = Or(x=w216, y="halt processor") -> (x .or. y?=w215:bool)
                    "IP address" <- w195
                    "ReA" <- w204
                    "RegB" <- w211
                    "RegC" <- w203
                    "FIFO size" <- w183
                    "RegD" <- w182
                  }
                  n224 = node-c288(w174) -> ()
                }
                frame True {
                }
              }
            }
          }
          frame #1 {
            n225 = local write "Run program"(FALSE ("Run program")) -> ()
          }
        }
      }
    }
  }
  n226 = while {
    tunnel: w1 -> [w636]
    stop <- FALSE stop-if-true
    n227 = flat-sequence {
      tunnel: w636 -> [w637]
      frame #0 {
        n228 = Wait on Occurrence(2:w637) -> ()  [unwired: 2 in, 1 out]
      }
      frame #1 {
        n229 = local read "AO7_pigeon"() -> (w638:i16)
        n230 = local write "AO7"(w638) -> ()
      }
    }
  }
  n231 = node-c288() -> (w8:T2)  [unwired: 1 in]
  n232 = while {
    shift-right: [w639] -> _
    shift-left: i16 0 -> [w640]
    stop <- FALSE stop-if-true
    n233 = case shown="False" "analog ramp on" {
      tunnel: [w643 w647] -> w639
      tunnel: w640 -> [w643 w644]
      frame False {
      }
      frame True {
        n234 = local read "analog ramp period"() -> (w646:i16)
        n235 = Less?(x=w644, y=w646) -> (x < y?=w645:bool)
        n236 = Increment(x=w644) -> (x+1=w648:i16)
        n237 = Not(x=w645) -> (.not. x?=w650:bool)
        n238 = Select(t=i16 0, s=w650, f=w648) -> (s? t:f=w647:i16)
        n239 = xnode "FPGA I/O Node"("Connector0/AO7"=w644) -> ()  [unwired: 1 in, 1 out]
        "Numeric" <- w644
      }
    }
  }
  n240 = while {
    stop <- FALSE stop-if-true
    n241 = xnode "FPGA I/O Node"() -> ("Connector0/AI0"=→"Connector0/AI0")  [unwired: 1 in, 1 out]
  }
  n242 = timed-loop {
    shift-right: [w654] -> _
    shift-left: u64 0 -> [w657]
    shift-right: [w656] -> _
    shift-left: TRUE -> [w655]
    timing: w8 -> [_]
    timing-out: [_] -> w7
    tunnel: [w656] -> _
    stop <- _ stop-if-true
    n243 = case shown="False" "square wave  on?" {
      tunnel: w657 -> [w659 w663]
      tunnel: [w658 w667] -> w656
      tunnel: w655 -> [w658 w666]
      tunnel: [w659 w664] -> w654
      frame False {
      }
      frame True {
        n244 = local read "square wave period"() -> (w662:i32)
        n245 = xnode "FPGA I/O Node"("Connector1/DIO6"=w666) -> ()  [unwired: 1 in, 1 out]
        n246 = Less?(x=w663, y=w662) -> (x < y?=w660:bool)
        n247 = Not(x=w660) -> (.not. x?=w661:bool)
        n248 = Increment(x=w663) -> (x+1=w669:u64)
        n249 = Not(x=w666) -> (.not. x?=w668:bool)
        n250 = Select(t=i16 0, s=w661, f=w669) -> (s? t:f=w664:u64)
        n251 = Greater Or Equal?(x=w664, y=w662) -> (x >= y?=w665:bool)
        n252 = Select(t=w668, s=w665, f=w666) -> (s? t:f=w667:bool)
      }
    }
  }
  n253 = node-c288(w7) -> ()
